vi "FreqSweepTest.vi"(0 "Signal Generator":refnum<class "Signal Generation.lvclass">, 1 "Scope":refnum<class "Scope.lvclass">, 2 "Amplitude (1)":dbl=0.5, 3 "Number of Steps (25)":i32=25, 4 "Input Channel (1)":dbl=1.0, 5 "error in (no error)":errorcluster, 6 "Waveform Function (1: Sine)":u16(ring)=1 items=["DC", "Sine", "Square", "Triangle", "Ramp", "Pulse", "Noise", "Sinc", "Negative Ramp", "Exponential Rise", "Exponential Fall", "Cardiac"], 7 "Start Frequency (1000)":dbl=1000.0, 9 "Stop Frequency (50000)":dbl=50000.0) -> (14 "Signal Generator Out":refnum<class "Signal Generation.lvclass">, 15 "Scope Out":refnum<class "Scope.lvclass">, 16 "Freq Amp Array":dbl[][](array[numeric])=[[1000.0, 25750.0, 50500.0, 75250.0, 100000.0], [6.881057614454697, 0.7762788757172112, 3.877116497313211, 5.5398055148465115, 8.936592894514183]], 19 "error out":errorcluster)   [LabVIEW 2010]
doc: "Executes a frequency sweep test by calling Generate Signal and ReadMaxAmp in a loop. The first frequency output is the start frequency and then the output frequency is incremented by (Stop Frequency - Start Frequency)/(Number of Steps). An Amplitude vs. Frequency array contains the test results."
uses:
  DSSP Modules/Output Classes/Signal Generation/Signal Generation.lvclass
  DSSP Modules/Input Classes/Scope/Scope.lvclass
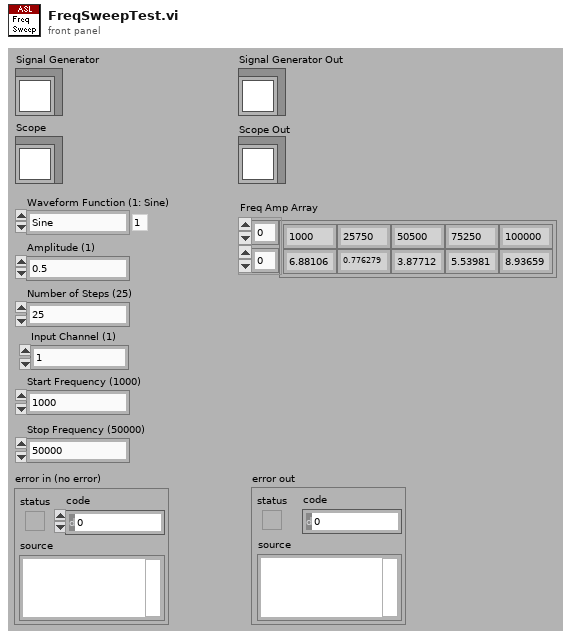
[diagram p1: front panel]
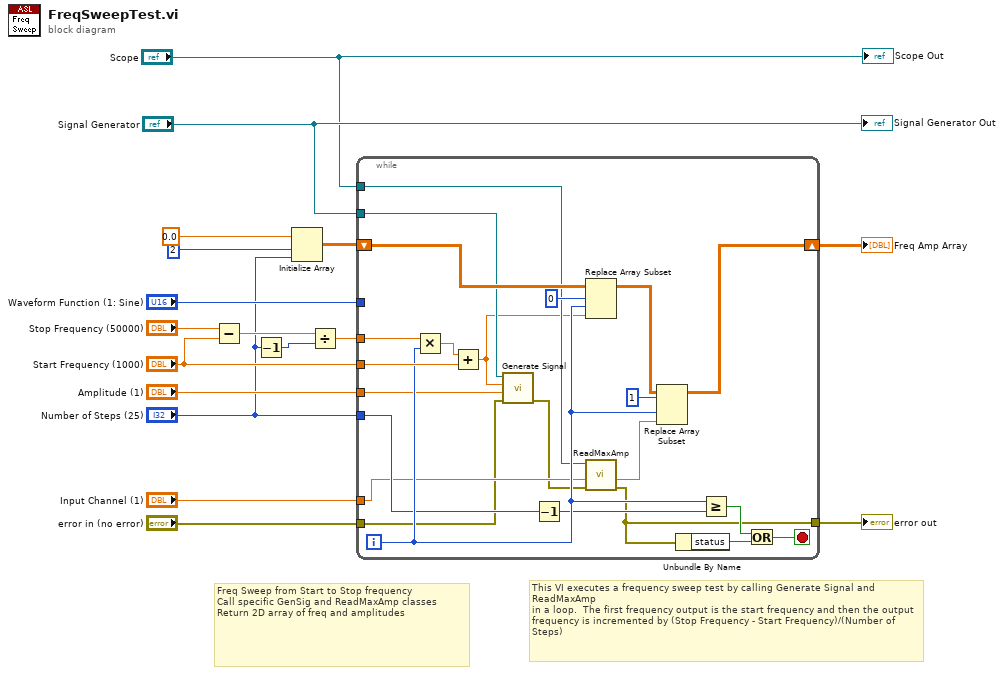
[diagram p0: block diagram]
diagram:
  # "This VI executes a frequency sweep test by calling Generate Signal and ReadMaxAmp\nin a loop.  The first frequency output is the start frequency and then the output frequency is incremented by (Stop Frequency - Start Frequency)/(Number of Steps)"
  # "Freq Sweep from Start to Stop frequency\nCall specific GenSig and ReadMaxAmp classes\nReturn 2D array of freq and amplitudes"
  n1 = Subtract(x="Stop Frequency (50000)", y="Start Frequency (1000)") -> (x-y=w13:dbl)
  n2 = Decrement(x="Number of Steps (25)") -> (x-1=w5:i32)
  n3 = Initialize Array(0.0 ("element"), 2 ("dimension size"), "Number of Steps (25)") -> (w8:dbl[][])
  n4 = Divide(x=w13, y=w5) -> (x/y=w11:dbl)
  n5 = while {
    tunnel: "error in (no error)" -> [w21]
    tunnel: "Waveform Function (1: Sine)" -> [_]
    tunnel: [w26] -> w4
    tunnel: "Input Channel (1)" -> [w24]
    tunnel: "Signal Generator" -> [w19]
    tunnel: "Scope" -> [w23]
    tunnel: "Start Frequency (1000)" -> [w39]
    tunnel: w11 -> [w38]
    tunnel: "Amplitude (1)" -> [w20]
    shift-right: [w33] -> w6
    shift-left: w8 -> [w37]
    tunnel: "Number of Steps (25)" -> [w28]
    i -> [w29]
    stop <- w31 stop-if-true
    n6 = Multiply(x=w38, y=w29) -> (x*y=w40:dbl)
    n7 = Add(x=w40, y=w39) -> (x+y=w18:dbl)
    n8 = call-dynamic "Generate Signal.vi"("error in (no error)"=w21, "Amplitude (1)"=w20, "Frequency (1000 Hz)"=w18, "Signal Generation In"=w19) -> ("error out"=w22:errorcluster)  [unwired: 7 out]
    n9 = Decrement(x=w28) -> (x-1=w27:i32)
    n10 = Replace Array Subset(array=w37, new element=w18, index (row)=0, index (col)=w29) -> (w35:dbl[][])
    n11 = call-dynamic "ReadMaxAmp.vi"("error in (no error)"=w22, "Channel"=w24, "Scope In"=w23) -> ("error out"=w26:errorcluster, "Amplitude"=w25:dbl)  [unwired: 7 out]
    n12 = Replace Array Subset(array=w35, new element=w25, index (row)=1, index (col)=w29) -> (w33:dbl[][])
    n13 = Unbundle By Name(w26) -> ("status"=w32:bool)
    n14 = Greater Or Equal?(x=w29, y=w27) -> (x >= y?=w30:bool)
    n15 = Or(x=w30, y=w32) -> (x .or. y?=w31:bool)
  }
  "Freq Amp Array" <- w6
  "error out" <- w4
  "Signal Generator Out" <- "Signal Generator"
  "Scope Out" <- "Scope"
